vi "Process--SMO.Example.vi"(8 "error in (no error)":errorcluster, 11 "SMO.Example in":refnum<class "SMO.Example.lvclass">) -> (0 "error out":errorcluster)   [LabVIEW 2013, in "SMO.Example.lvclass"]
uses:
  SMO.Example.lvclass
  src/SMO/SMO.lvclass
panel:
  out "Flow 2":dbl
  out "Flow 1":dbl
  in  "Pump State":bool
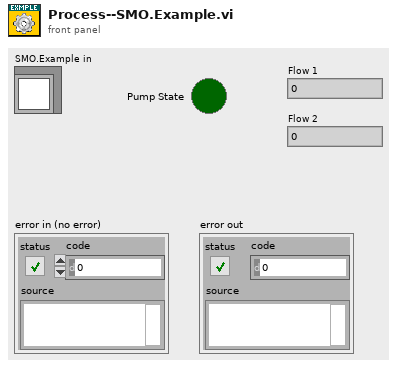
[diagram p1: front panel]
types:
  T1 = enum32{"invalid app kind", "Development System", "Run Time System", "Student Edition", "Embedded LabVIEW", "Evaluation", "Custom"}
  T2 = enum32{"Invalid", "Standard", "Closed", "Hidden", "Minimized", "Maximized"}
  T3 = cluster{"Core":cluster{"Current VI Reference":refnum<vi>, "Close Panel on Exit?":bool, "error":errorcluster, "Standalone":bool}, "Self Ref":refnum<class "SMO.Example.lvclass">, "Your string data":string, "Pump State":bool, "Valve 1 State":bool, "Flow 1 Actual":dbl, "Flow 2 Actual":dbl, "Flow 1 Target":dbl, "Flow 2 Target":dbl}
  T4 = typedef "SMO.lvclass/SMOState --Enum.ctl" = enum16{"unknown", "Created", "Started", "Stopped"}
  T5 = cluster{"Current VI Reference":refnum<vi>, "Close Panel on Exit?":bool, "error":errorcluster, "Standalone":bool}
  T6 = typedef "SMO.lvclass/Protected Events.ctl" = cluster{"StopProcesses":refnum<user-event>, "AbortProcesses":refnum<user-event>, "Config Changed":refnum<user-event>, "Dependency":refnum<user-event>}
  T7 = typedef "SMO.Example.lvclass/ProtectedEvents--Cluster.ctl" = cluster{"API_Template":refnum<user-event>, "PumpState":refnum<user-event>, "Valve State":refnum<user-event>}
  T8 = typedef "SMO.Example.lvclass/PublicEvents--Cluster.ctl" = cluster{"Data Changed":refnum<user-event>, "State Changed":refnum<user-event>}
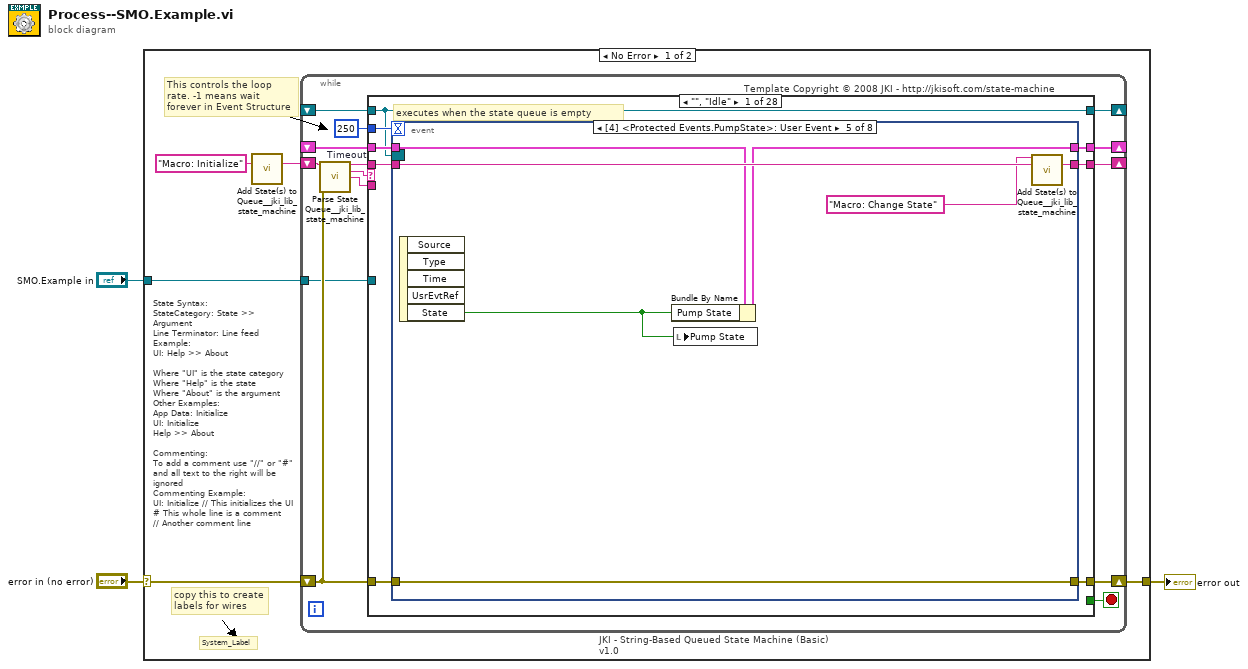
[diagram p0: block diagram]
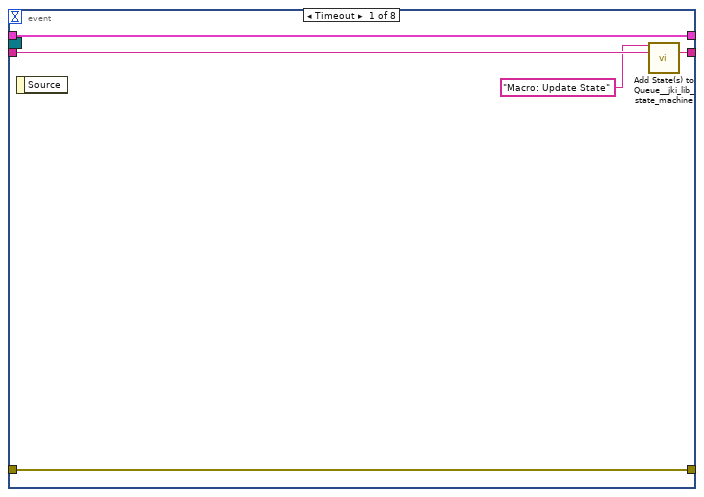
[diagram p2: hidden frame]
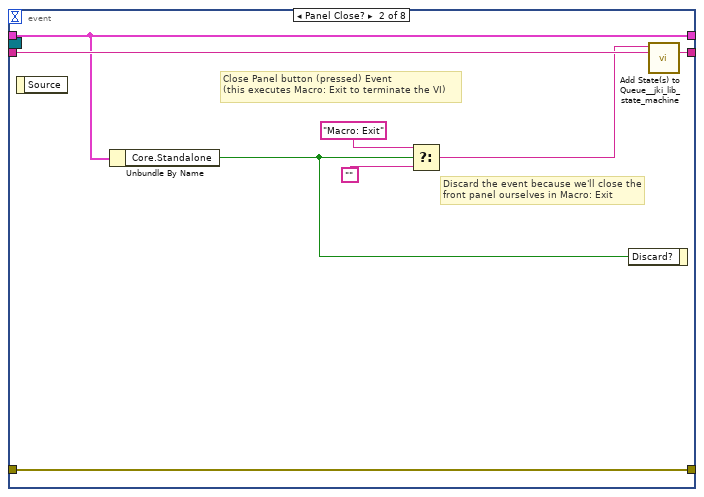
[diagram p3: hidden frame]
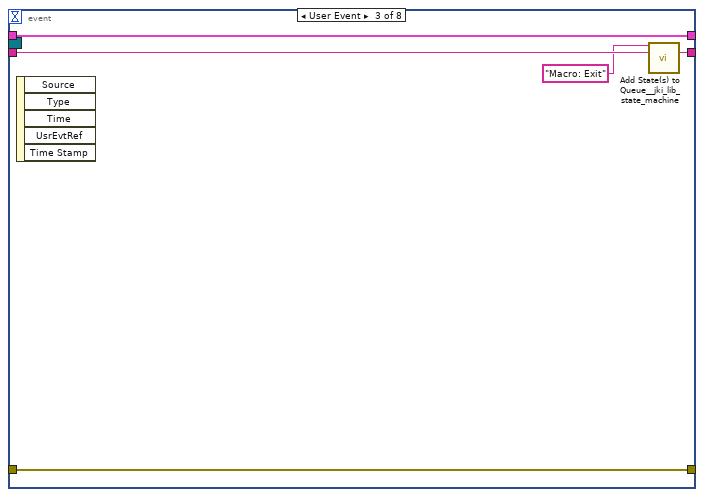
[diagram p4: hidden frame]
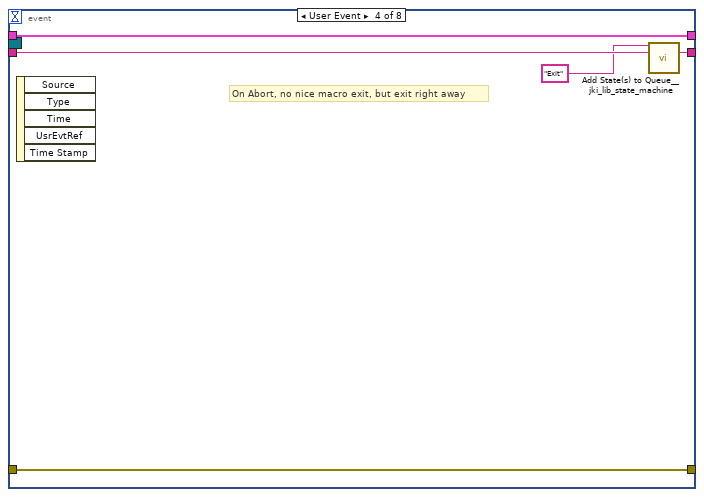
[diagram p5: hidden frame]
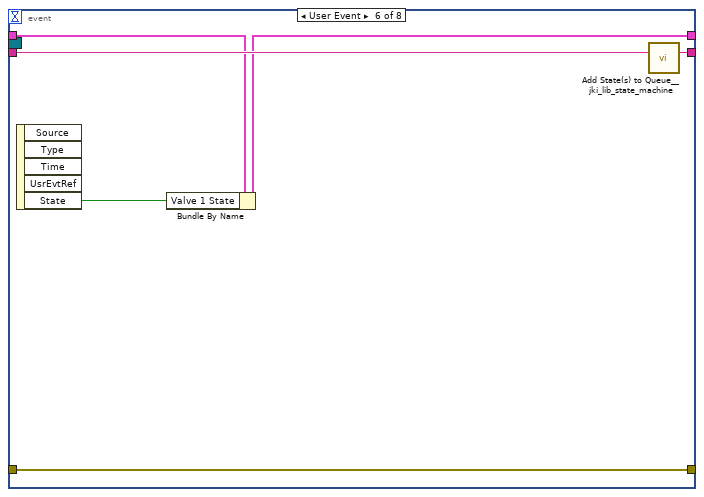
[diagram p6: hidden frame]
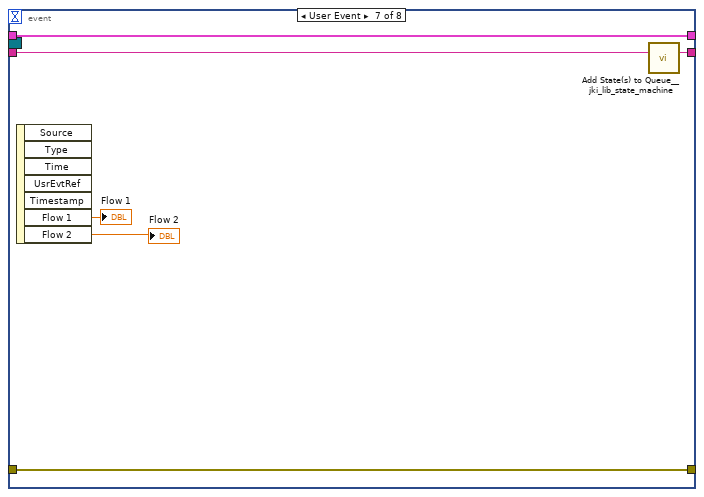
[diagram p7: hidden frame]
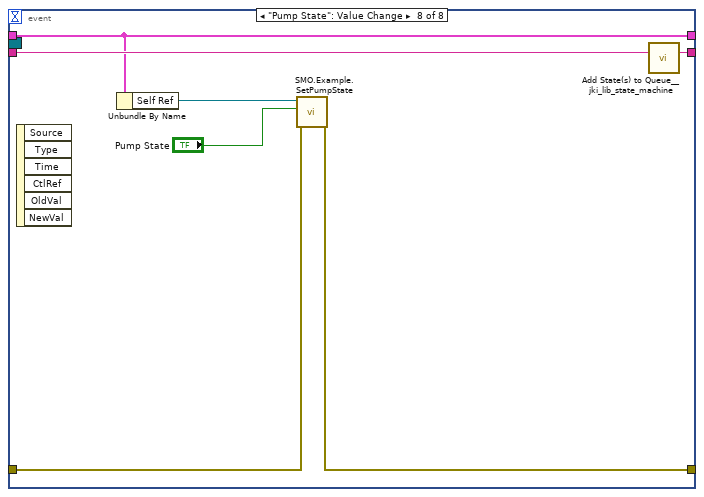
[diagram p8: hidden frame]
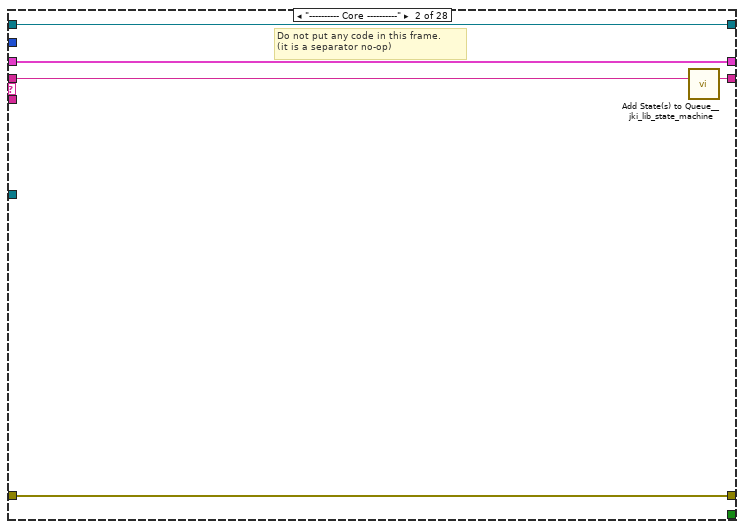
[diagram p9: hidden frame]
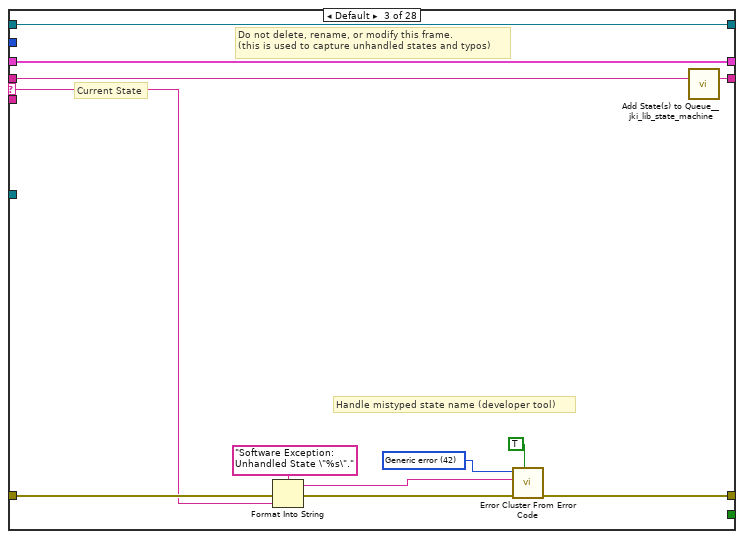
[diagram p10: hidden frame]
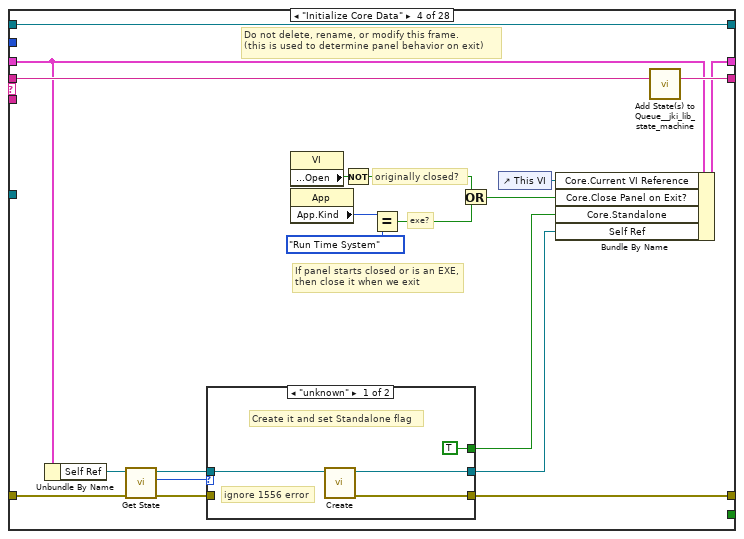
[diagram p11: hidden frame]
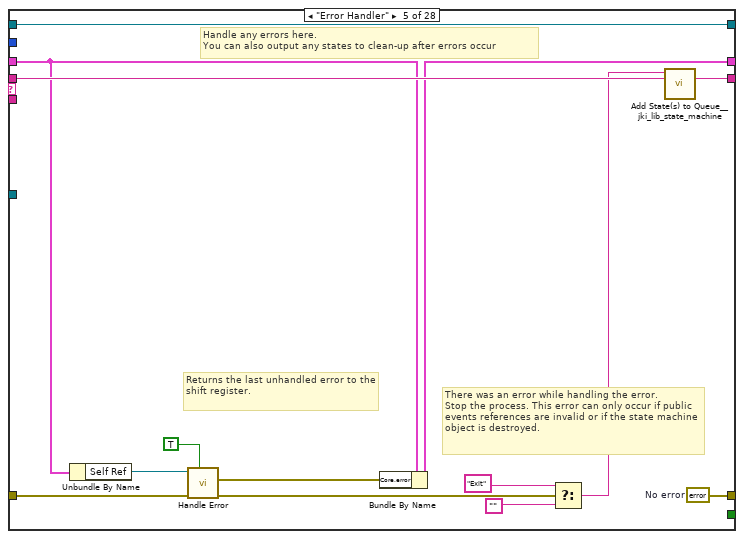
[diagram p13: hidden frame]
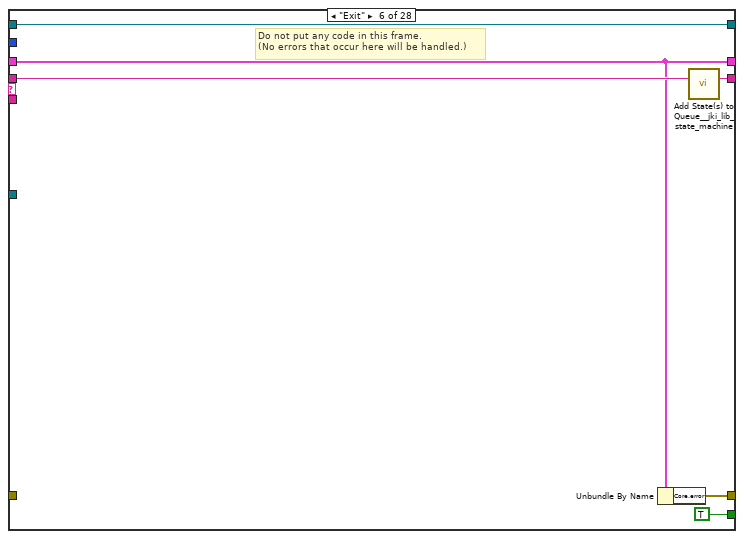
[diagram p14: hidden frame]
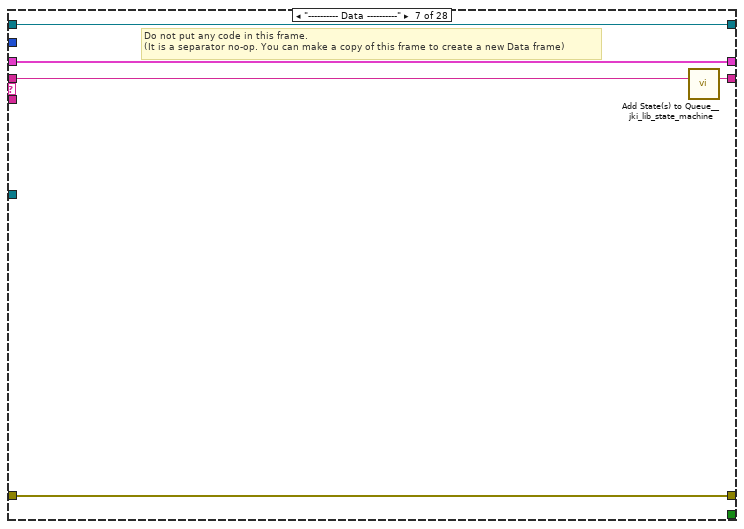
[diagram p15: hidden frame]
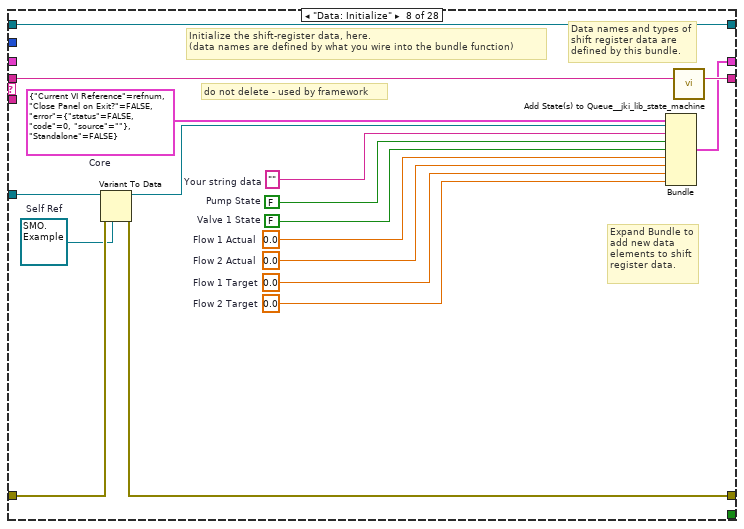
[diagram p16: hidden frame]
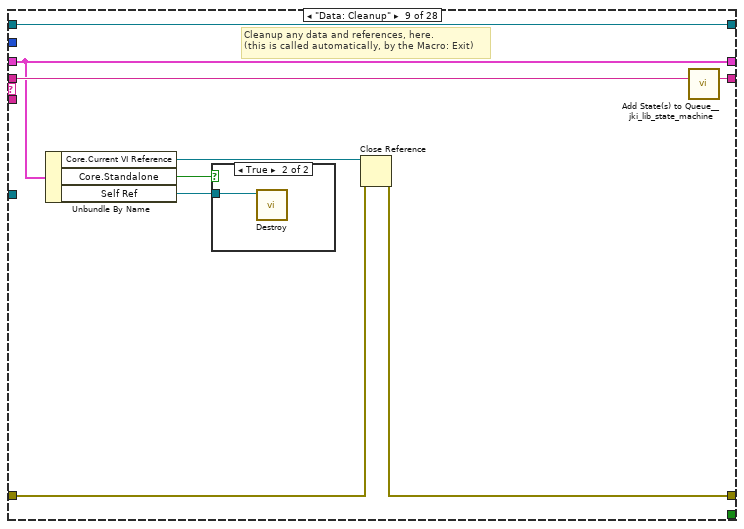
[diagram p17: hidden frame]
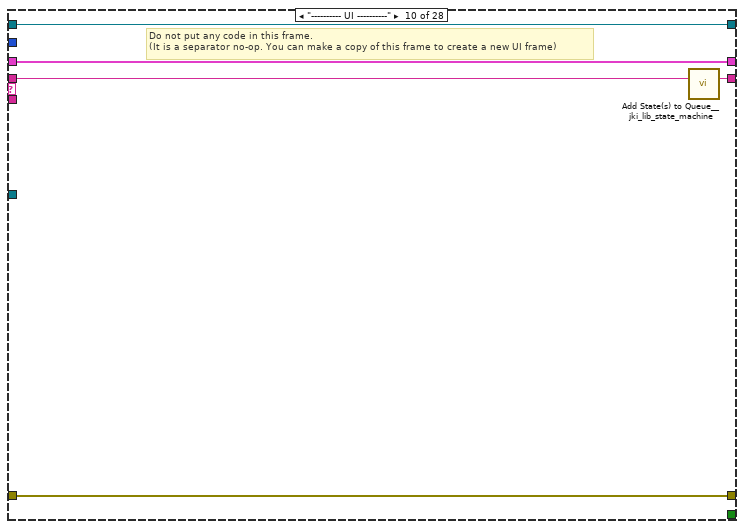
[diagram p19: hidden frame]
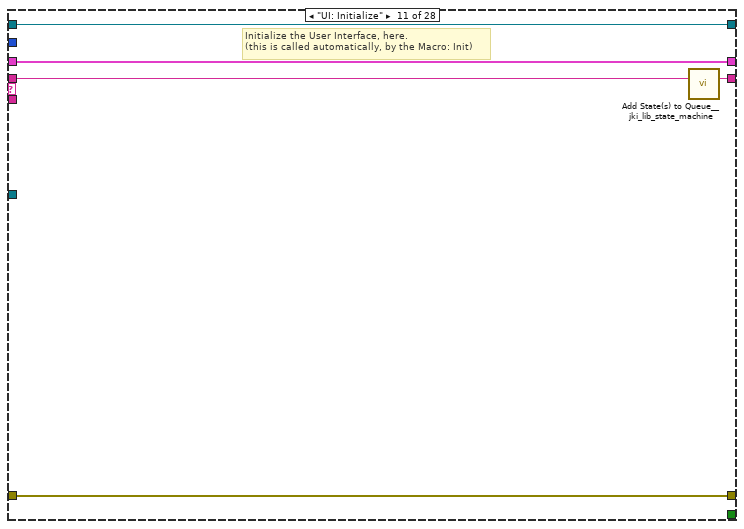
[diagram p20: hidden frame]
diagram:
  n1 = case shown="No Error" "error in (no error)" {
    selector: "error in (no error)" -> [w5 w378]
    tunnel: "SMO.Example in" -> [w6 _]
    tunnel: [w4 w378] -> w3
    frame No Error {
      # "State Syntax:\nStateCategory: State >> Argument\nLine Terminator: Line feed\nExample:\nUI: Help >> About\n\nWhere \"UI\" is the state category\nWhere \"Help\" is the state\nWhere \"About\" is the argument\nOther Examples:\nApp Data: Initialize\nUI: Initialize\nHelp >> About\n\nCommenting:\nTo add a comment use \"//\" or \"#\" and all text to the right will be ignored\nCommenting Example:\nUI: Initialize // This initializes the UI\n# This whole line is a comment\n// Another comment line"
      # "copy this to create labels for wires"
      # "This controls the loop rate. -1 means wait forever in Event Structure"
      # "System_Label"
      n2 = call <vilib>:"Add State(s) to Queue__jki_lib_state_machine.vi"("State(s) in (\"\")"="Macro: Initialize") -> ("States Out"=w8:string)  [unwired: 14 in]
      n3 = while "JKI - String-Based Queued State Machine (Basic) v1.0" {
        shift-right: [w15] -> _
        shift-left: _ -> [w14]
        shift-right: [w18] -> w4
        shift-left: w5 -> [w12]
        shift-right: [w17] -> _
        shift-left: w8 -> [w19]
        tunnel: w6 -> [w11]
        shift-right: [w10] -> _
        shift-left: _ -> [w9]
        stop <- w16 stop-if-true
        w13 = 250  # Timeout
        # "Template Copyright © 2008 JKI - http://jkisoft.com/state-machine"
        n4 = call <vilib>:"Parse State Queue__jki_lib_state_machine.vi"("State Queue"=w19, "Error In (no error)"=w12) -> ("Remaining States"=w21:string, "Current State"=w22:string, "Arguments"=w20:string)  [unwired: 11 in]
        n5 = case shown="\"\", \"Idle\"" w22 {
          selector: w22 -> [_ _ w86 _ _ _ _ _ _ _ _ _ _ _ _ _ _ _ _ _ _ _ _ _ _ _ _ _]
          tunnel: w21 -> [w30 w84 w90 w116 w136 w142 w147 w164 w173 w179 w184 w189 w197 w229 w238 w244 w250 w261 w266 w275 w288 w303 w309 w314 w324 w360 w369 w377]
          tunnel: w20 -> [_ _ _ _ _ _ _ _ _ _ _ _ w190 _ _ _ _ _ _ _ _ _ _ _ _ _ _ _]
          tunnel: w14 -> [w28 w81 w88 w104 w127 w138 w144 _ w168 w176 w182 w187 w195 w226 w234 w241 w247 w252 w263 w272 w285 w301 w307 w312 w318 w356 w366 w374]
          tunnel: [w27 w82 w92 w100 w124 w137 w145 w159 w169 w177 w181 w185 w191 w227 w236 w242 w248 w259 w264 w269 w286 w295 w305 w310 w319 w357 w363 w370] -> w18
          tunnel: w12 -> [w26 w82 w91 w103 w128 _ w145 w160 w170 w177 w181 w185 w192 w227 w236 w242 w248 w259 w264 w270 w286 w297 w305 w310 w319 w357 w364 w371]
          tunnel: [w29 w83 w89 w115 w135 w141 w146 w163 w172 w178 w183 w188 w196 w228 w237 w243 w249 w260 w265 w274 w287 w302 w308 w313 w323 w359 w368 w376] -> w17
          tunnel: [_ _ _ _ _ TRUE _ _ _ _ _ _ _ _ _ _ _ _ _ _ _ _ _ _ _ _ _ _] -> w16
          tunnel: [w25 w81 w88 w114 w126 w138 w144 w162 w168 w176 w182 w187 w195 w226 w234 w241 w247 w252 w263 w272 w285 w301 w307 w312 w317 w355 w366 w374] -> w15
          tunnel: w13 -> [w24 _ _ _ _ _ _ _ _ _ _ _ _ _ _ _ _ _ _ _ _ _ _ _ _ _ _ _]
          tunnel: w11 -> [_ _ _ _ _ _ _ w157 _ _ _ _ _ _ _ _ _ _ _ _ _ _ _ _ _ _ _ _]
          tunnel: [w23 w80 w85 w107 w134 w139 w143 w155 w167 w175 w180 w186 w194 w225 w235 w240 w246 w253 w262 w273 w284 w299 w306 w311 w322 w358 w367 w375] -> w10
          tunnel: w9 -> [w23 w80 w85 w107 w134 w139 w143 w155 w167 w175 w180 w186 w194 w225 w235 w240 w246 w253 w262 w273 w284 _ w306 w311 w322 w358 w367 w375]
          frame "", "Idle" {
            # "executes when the state queue is empty"
            n6 = event shown="[4] <Protected Events.PumpState>: User Event" {
              selector: w23 -> [_ _ _ _ _ _ _ _]
              dyn-events: _ -> [_ _ _ _ _ _ _ _]
              timeout: w24 -> [_ _ _ _ _ _ _ _]
              tunnel: w30 -> [w35 w43 w48 w53 w60 w66 w72 w79]
              tunnel: [w34 w42 w47 w52 w59 w65 w71 w78] -> w29
              tunnel: w28 -> [w32 w40 w45 w50 w57 w63 w69 w77]
              tunnel: [w33 w41 w46 w51 w58 w64 w70 w73] -> w27
              tunnel: w26 -> [w33 w41 w46 w51 w58 w64 w70 w74]
              tunnel: [w32 w40 w45 w50 w56 w62 w69 w77] -> w25
              event Timeout {
                n7 = event-data() -> ()  [unwired: 1 in, 1 out]
                n8 = call <vilib>:"Add State(s) to Queue__jki_lib_state_machine.vi"("State(s) in Front (\"\")"="Macro: Update State", "State(s) in (\"\")"=w35) -> ("States Out"=w34:string)  [unwired: 13 in]
              }
              event Panel Close? {
                # "Discard the event because we'll close the front panel ourselves in Macro: Exit"
                # "Close Panel button (pressed) Event\n(this executes Macro: Exit to terminate the VI)"
                n9 = event-data() -> ()  [unwired: 1 in, 1 out]
                n10 = Unbundle By Name(w40) -> ("Core.Standalone"=w36:bool)
                n11 = Select(t="Macro: Exit", s=w36, f="") -> (s? t:f=w37:string)
                n12 = event-data("Discard?"=w36) -> ()  [unwired: 1 in, 1 out]
                n13 = call <vilib>:"Add State(s) to Queue__jki_lib_state_machine.vi"("State(s) in Front (\"\")"=w37, "State(s) in (\"\")"=w43) -> ("States Out"=w42:string)  [unwired: 13 in]
              }
              event User Event {
                n14 = event-data() -> ()  [unwired: 1 in, 5 out]
                n15 = call <vilib>:"Add State(s) to Queue__jki_lib_state_machine.vi"("State(s) in Front (\"\")"="Macro: Exit", "State(s) in (\"\")"=w48) -> ("States Out"=w47:string)  [unwired: 13 in]
              }
              event User Event {
                # "On Abort, no nice macro exit, but exit right away"
                n16 = event-data() -> ()  [unwired: 1 in, 5 out]
                n17 = call <vilib>:"Add State(s) to Queue__jki_lib_state_machine.vi"("State(s) in Front (\"\")"="Exit", "State(s) in (\"\")"=w53) -> ("States Out"=w52:string)  [unwired: 13 in]
              }
              event User Event {
                n18 = event-data() -> ("State"=w54:bool)  [unwired: 1 in, 4 out]
                n19 = Bundle By Name(cluster=w57, "Pump State"=w54) -> (w56:T3)
                n20 = local write "Pump State"(w54) -> ()
                n21 = call <vilib>:"Add State(s) to Queue__jki_lib_state_machine.vi"("State(s) in Front (\"\")"="Macro: Change State", "State(s) in (\"\")"=w60) -> ("States Out"=w59:string)  [unwired: 13 in]
              }
              event User Event {
                n22 = event-data() -> ("State"=w61:bool)  [unwired: 1 in, 4 out]
                n23 = Bundle By Name(cluster=w63, "Valve 1 State"=w61) -> (w62:T3)
                n24 = call <vilib>:"Add State(s) to Queue__jki_lib_state_machine.vi"("State(s) in (\"\")"=w66) -> ("States Out"=w65:string)  [unwired: 14 in]
              }
              event User Event {
                n25 = event-data() -> ("Flow 1"=→"Flow 1":dbl, "Flow 2"=→"Flow 2":dbl)  [unwired: 1 in, 5 out]
                n26 = call <vilib>:"Add State(s) to Queue__jki_lib_state_machine.vi"("State(s) in (\"\")"=w72) -> ("States Out"=w71:string)  [unwired: 14 in]
              }
              event "Pump State": Value Change {
                n27 = event-data() -> ()  [unwired: 1 in, 6 out]
                n28 = Unbundle By Name(w77) -> ("Self Ref"=w76:refnum<class "SMO.Example.lvclass">)
                n29 = call "SMO.Example.SetPumpState.vi"("error in (no error)"=w74, "Pump State"="Pump State", "SMO.Example"=w76) -> ("error out"=w73:errorcluster)  [unwired: 7 in, 1 out]
                n30 = call <vilib>:"Add State(s) to Queue__jki_lib_state_machine.vi"("State(s) in (\"\")"=w79) -> ("States Out"=w78:string)  [unwired: 14 in]
              }
            }
          }
          frame "---------- Core ----------" {
            # "Do not put any code in this frame.\n(it is a separator no-op)"
            n31 = call <vilib>:"Add State(s) to Queue__jki_lib_state_machine.vi"("State(s) in (\"\")"=w84) -> ("States Out"=w83:string)  [unwired: 14 in]
          }
          frame Default {
            w95 = 42 items=["No error", "Argument error", "Memory is full", "Out of zone", "End of file", "File already open", "Generic file I/O error", "File not found", "File permission error", "Disk is full", "Duplicate path", "Too many files open", "System feature not enabled", "Resource file not found", "Cannot add resource", "Resource not found", "Image not found", "Image memory error", "Pen does not exist", "Config type invalid", "Config token not found", "Config parse error", "Config memory error", "Bad external code format", "Bad external code offset", "External code not present", "Null window", "Destroy window error", "Null menu", "Print aborted", "Bad print record", "Print driver error", "Windows error during printing", "Memory error during printing", "Print dialog error", "Generic print error", "Invalid device refnum", "Device not found", "Device parameter error", "Device unit error", "Cannot open device", "Device call aborted", "Generic error", "Cancelled by user", "Object ID too low", "Object ID too high", "Object not in heap", "Unknown heap", "Unknown object (invalid DefProc)", "Unknown object (DefProc not in table)", "Message out of range", "Invalid (null) method", "Unknown message", "Manager call not supported", "Bad address", "Network operation in progress", "Network operation timed out", "Connection is busy", "Network attribute not supported", "Network error", "Address in use", "System out of memory", "Connection aborted", "Connection refused", "Not connected", "Already connected", "Connection closed", "Initialization error (interapplication manager)", "Bad occurrence", "Wait on unbound occurrence handler", "Occurrence queue overflow", "Datalog type conflict", "Unused", "Unrecognized type (interapplication manager)", "Memory corrupt", "Failed to make temporary DLL", "Old CIN version", "Drag socket not found", "Failed to load drop-object", "Failed to register OLE object", "Failed to release OLE object", "Format specifier type mismatch", "Unknown format specifier", "Too few format specifiers", "Too many format specifiers", "Scan failed", "Newer CIN version", "Error converting to variant", "Runtime menu error", "Password tampered", "Variant attribute not found", "Incompatible variant data type", "Event data is not available", "Event Store is not present", "Occurrence is not found", "Event Queue is not created", "Event info is not available", "Refnum passed is NULL", "Error retrieving Class GUID", "Error retrieving CoClass GUID", "Error retrieving TypeLib GUID.", "Bad built application magic bytes.", "Specific driver is different from the specific driver associated with the Logical Name.", "There is no session opened to the class driver.", "Max Error", "MAX - Error with config objects", "MAX - Error loading configuration", "MAX - Group not supported"]
            # "Current State"
            # "Do not delete, rename, or modify this frame.\n(this is used to capture unhandled states and typos)"
            # "Handle mistyped state name (developer tool)"
            n32 = Format Into String(format string="Software Exception: Unhandled State \"%s\"." ("message"), error in=w91, w86) -> (resulting string=w94:string, error out=w93:errorcluster)  [unwired: 1 in]
            n33 = call <vilib>:"Error Cluster From Error Code.vi"("show call chain? (False)"=TRUE, "error in (no error)"=w93, "error message (\"\")"=w94, "error code (0)"=w95) -> ("error out"=w92:errorcluster)  [unwired: 5 in]
            n34 = call <vilib>:"Add State(s) to Queue__jki_lib_state_machine.vi"("State(s) in (\"\")"=w90) -> ("States Out"=w89:string)  [unwired: 14 in]
          }
          frame "Initialize Core Data" {
            # "Do not delete, rename, or modify this frame.\n(this is used to determine panel behavior on exit)"
            # "originally closed?"
            # "exe?"
            # "If panel starts closed or is an EXE, then close it when we exit"
            n35 = Unbundle By Name(w104) -> ("Self Ref"=w105:refnum<class "SMO.Example.lvclass">)
            n36 = call "Get State.vi"("error in (no error)"=w103, "SMO"=w105) -> ("error out"=w101:errorcluster, "SMO State"=w102:T4, "SMO out"=w98:refnum<class "SMO.Example.lvclass">)  [unwired: 7 in]
            n37 = case shown="\"unknown\"" w102 {
              tunnel: w101 -> [_ w122]
              tunnel: [w119 w122] -> w100
              tunnel: [TRUE _] -> w99
              tunnel: w98 -> [w118 w121]
              tunnel: [w117 w121] -> w97
              frame "unknown" {
                # "ignore 1556 error"
                # "Create it and set Standalone flag"
                n38 = call "Create.vi"("SMO"=w118) -> ("error out"=w119:errorcluster, "SMO out"=w117:refnum<class "SMO.Example.lvclass">)  [unwired: 8 in, 1 out]
              }
              frame Default {
              }
            }
            n39 = property class="VI"() -> ("Front Panel.Open"=w113:bool)  [unwired: 2 in, 2 out]
            n40 = property class="App"() -> ("App.Kind"=w112:T1)  [unwired: 2 in, 2 out]
            n41 = Not(x=w113) -> (.not. x?=w110:bool)
            n42 = Equal?(x=w112, y=T1."Run Time System" ("Application:Kind")) -> (x = y?=w109:bool)
            n43 = Or(x=w110, y=w109) -> (x .or. y?=w108:bool)
            n44 = control-ref of="This VI"() -> (w106:refnum<vi>)
            n45 = Bundle By Name(cluster=w104, "Core.Current VI Reference"=w106, "Core.Close Panel on Exit?"=w108, "Core.Standalone"=w99, "Self Ref"=w97) -> (w114:T3)
            n46 = call <vilib>:"Add State(s) to Queue__jki_lib_state_machine.vi"("State(s) in (\"\")"=w116) -> ("States Out"=w115:string)  [unwired: 14 in]
          }
          frame "Error Handler" {
            w124 = errorcluster {"status"=FALSE, "code"=0, "source"=""}  # No error
            # "Returns the last unhandled error to the shift register."
            # "There was an error while handling the error.\nStop the process. This error can only occur if public events references are invalid or if the state machine object is destroyed."
            # "Handle any errors here.\nYou can also output any states to clean-up after errors occur"
            n47 = Unbundle By Name(w127) -> ("Self Ref"=w129:refnum<class "SMO.Example.lvclass">)
            n48 = call-dynamic "Handle Error.vi"("Stop on Unhandled Error (T)"=TRUE, "error in"=w128, "SMO"=w129) -> ("handling error"=w131:errorcluster, "Unhandled error"=w130:errorcluster)  [unwired: 6 in, 1 out]
            n49 = Bundle By Name(cluster=w127, "Core.error"=w130) -> (w126:T3)
            n50 = Select(t="Exit", s=w131, f="") -> (s? t:f=w125:string)
            n51 = call <vilib>:"Add State(s) to Queue__jki_lib_state_machine.vi"("State(s) in Front (\"\")"=w125, "State(s) in (\"\")"=w136) -> ("States Out"=w135:string)  [unwired: 13 in]
          }
          frame "Exit" {
            # "Do not put any code in this frame.\n(No errors that occur here will be handled.)"
            n52 = Unbundle By Name(w138) -> ("Core.error"=w137:errorcluster)
            n53 = call <vilib>:"Add State(s) to Queue__jki_lib_state_machine.vi"("State(s) in (\"\")"=w142) -> ("States Out"=w141:string)  [unwired: 14 in]
          }
          frame "---------- Data ----------" {
            # "Do not put any code in this frame.\n(It is a separator no-op. You can make a copy of this frame to create a new Data frame)"
            n54 = call <vilib>:"Add State(s) to Queue__jki_lib_state_machine.vi"("State(s) in (\"\")"=w147) -> ("States Out"=w146:string)  [unwired: 14 in]
          }
          frame "Data: Initialize" {
            w148 = T5 {"Current VI Reference"=refnum, "Close Panel on Exit?"=FALSE, "error"={"status"=FALSE, "code"=0, "source"=""}, "Standalone"=FALSE}  # Core
            w149 = 0.0  # Flow 2 Target
            w150 = 0.0  # Flow 1 Target
            w151 = 0.0  # Flow 2 Actual
            w152 = 0.0  # Flow 1 Actual
            w153 = FALSE  # Valve 1 State
            w154 = FALSE  # Pump State
            w158 = refnum<class "SMO.Example.lvclass"> refnum  # Self Ref
            w161 = ""  # Your string data
            # "do not delete - used by framework"
            # "Expand Bundle to add new data elements to shift register data."
            # "Data names and types of shift register data are defined by this bundle."
            # "Initialize the shift-register data, here.\n(data names are defined by what you wire into the bundle function)"
            n55 = Variant To Data(error in=w160, type=w158, Variant=w157) -> (data=w156:refnum<class "SMO.Example.lvclass">, error out=w159:errorcluster)
            n56 = Bundle("Core"=w148, "Self Ref"=w156, "Your string data"=w161, "Pump State"=w154, "Valve 1 State"=w153, "Flow 1 Actual"=w152, "Flow 2 Actual"=w151, "Flow 1 Target"=w150, "Flow 2 Target"=w149) -> (w162:T3)  [unwired: 1 in]
            n57 = call <vilib>:"Add State(s) to Queue__jki_lib_state_machine.vi"("State(s) in (\"\")"=w164) -> ("States Out"=w163:string)  [unwired: 14 in]
          }
          frame "Data: Cleanup" {
            # "Cleanup any data and references, here.\n(this is called automatically, by the Macro: Exit)"
            n58 = Unbundle By Name(w168) -> ("Core.Current VI Reference"=w171:refnum<vi>, "Core.Standalone"=w166:bool, "Self Ref"=w165:refnum<class "SMO.Example.lvclass">)
            n59 = case shown="True" w166 {
              tunnel: w165 -> [_ w174]
              frame False {
              }
              frame True {
                n60 = call "Destroy.vi"("SMO"=w174) -> ()  [unwired: 10 in, 1 out]
              }
            }
            n61 = Close Reference(reference=w171, error in (no error)=w170) -> (error out=w169:errorcluster)
            n62 = call <vilib>:"Add State(s) to Queue__jki_lib_state_machine.vi"("State(s) in (\"\")"=w173) -> ("States Out"=w172:string)  [unwired: 14 in]
          }
          frame "---------- UI ----------" {
            # "Do not put any code in this frame.\n(It is a separator no-op. You can make a copy of this frame to create a new UI frame)"
            n63 = call <vilib>:"Add State(s) to Queue__jki_lib_state_machine.vi"("State(s) in (\"\")"=w179) -> ("States Out"=w178:string)  [unwired: 14 in]
          }
          frame "UI: Initialize" {
            # "Initialize the User Interface, here.\n(this is called automatically, by the Macro: Init)"
            n64 = call <vilib>:"Add State(s) to Queue__jki_lib_state_machine.vi"("State(s) in (\"\")"=w184) -> ("States Out"=w183:string)  [unwired: 14 in]
          }
          frame "UI: Cursor Set" {
            # "Deleted Cursor Busy code\nto make process RT-compatible"
            # "Initialize the User Interface, here.\n(this is called automatically, by the Macro: Init)"
            n65 = call <vilib>:"Add State(s) to Queue__jki_lib_state_machine.vi"("State(s) in (\"\")"=w189) -> ("States Out"=w188:string)  [unwired: 14 in]
          }
          frame "UI: Front Panel State" {
            # "Argument"
            # "Set Front Panel Open or Closed\n(Usage: \"UI: Front Panel State >> Open|Close\")"
            n66 = Unbundle By Name(w195) -> ("Core.Current VI Reference"=w193:refnum<vi>)
            n67 = disable-structure shown="Default" {
              disable-tunnel: w192 -> [w201 w224]
              disable-tunnel: [w200 w224] -> w191
              disable-tunnel: w193 -> [w199 _]
              disable-tunnel: w190 -> [w198 _]
              frame condition #0 (active) {
                n68 = case shown="\"Open\"" w198 {
                  tunnel: w201 -> [w205 w218]
                  tunnel: [w207 w219] -> w200
                  tunnel: w199 -> [w206 w216]
                  frame "Open" {
                    # "Open FP if not open or invalid"
                    n69 = property class="VI"(reference=w206, error in=w205) -> (reference out=w203:refnum<vi>, error out=w204:errorcluster, "FP.State"=w202:T2)
                    n70 = case shown="Default" w202 {
                      tunnel: [w210 w213] -> w207
                      tunnel: w204 -> [w209 w213]
                      tunnel: w203 -> [w208 _]
                      frame Default {
                        n71 = invoke class="VI" method="FP.Open"(reference=w208, error in=w209, "Activate"=TRUE, "State"=T2."Standard") -> (error out=w210:errorcluster)  [unwired: 1 in, 4 out]
                      }
                      frame "Invalid", "Standard" {
                      }
                    }
                  }
                  frame "Close", Default {
                    # "Close FP is not Closed or Invalid"
                    n72 = property class="VI"(reference=w216, error in=w218) -> (reference out=w215:refnum<vi>, error out=w217:errorcluster, "FP.State"=w214:T2)
                    n73 = case shown="Default" w214 {
                      tunnel: [w220 w223] -> w219
                      tunnel: w217 -> [w220 w222]
                      tunnel: w215 -> [_ w221]
                      frame "Invalid", "Closed" {
                      }
                      frame Default {
                        n74 = invoke class="VI" method="FP.Close"(reference=w221, error in=w222) -> (error out=w223:errorcluster)  [unwired: 1 in, 2 out]
                      }
                    }
                  }
                }
              }
              frame condition #1 {
              }
            }
            n75 = call <vilib>:"Add State(s) to Queue__jki_lib_state_machine.vi"("State(s) in (\"\")"=w197) -> ("States Out"=w196:string)  [unwired: 14 in]
          }
          frame "---------- Macro ----------" {
            # "Do not put any code in this frame.\n(It is a separator no-op. You can make a copy of this frame to create a new Macro frame)"
            n76 = call <vilib>:"Add State(s) to Queue__jki_lib_state_machine.vi"("State(s) in (\"\")"=w229) -> ("States Out"=w228:string)  [unwired: 14 in]
          }
          frame "Macro: Initialize" {
            w232 = "UI: Initialize\n//UI: Front Panel State >> Open"  # UI: Initialize //UI: Front Panel State >> Open
            # "Initialization Macro\n(This is called once, when the VI starts)"
            n77 = call <vilib>:"Add State(s) to Queue__jki_lib_state_machine.vi"("State(s) in Front (\"\")"="Data: Initialize\nInitialize Core Data\nEvents: Register", "State(s) in (\"\")"="Process: Sync", "State(s) at Back (\"\")"=w232) -> ("States Out"=w231:string)  [unwired: 12 in]
            n78 = call <vilib>:"Add State(s) to Queue__jki_lib_state_machine.vi"("State(s) in Front (\"\")"=w231, "State(s) in (\"\")"=w238) -> ("States Out"=w237:string)  [unwired: 13 in]
          }
          frame "Macro: Update State" {
            n79 = call <vilib>:"Add State(s) to Queue__jki_lib_state_machine.vi"("State(s) in Front (\"\")"="Action: Determine Flow Targets\nAction: Determine Actual Flow\nAction: Update State", "State(s) in (\"\")"=w244) -> ("States Out"=w243:string)  [unwired: 13 in]
          }
          frame "Macro: Change State" {
            n80 = call <vilib>:"Add State(s) to Queue__jki_lib_state_machine.vi"("State(s) in Front (\"\")"="Action: Change State\nAction: Update State", "State(s) in (\"\")"=w250) -> ("States Out"=w249:string)  [unwired: 13 in]
          }
          frame "Macro: Exit" {
            # "Exit Macro\n(This is called once, when the VI exits)"
            n81 = Unbundle By Name(w252) -> ("Core.Close Panel on Exit?"=w258:bool)
            n82 = Select(t="//UI: Front Panel State >> Close", s=w258, f="") -> (s? t:f=w255:string)
            n83 = call <vilib>:"Add State(s) to Queue__jki_lib_state_machine.vi"("State(s) in (\"\")"=w255, "State(s) at Back (\"\")"="Data: Cleanup\nEvents: Unregister\nProcess: Sync\nExit") -> ("States Out"=w254:string)  [unwired: 13 in]
            n84 = call <vilib>:"Add State(s) to Queue__jki_lib_state_machine.vi"("State(s) in Front (\"\")"=w254, "State(s) in (\"\")"=w261) -> ("States Out"=w260:string)  [unwired: 13 in]
          }
          frame "---------- Process ----------" {
            # "Template Separator\n(You can make a copy of, or modify, this frame)"
            n85 = call <vilib>:"Add State(s) to Queue__jki_lib_state_machine.vi"("State(s) in (\"\")"=w266) -> ("States Out"=w265:string)  [unwired: 14 in]
          }
          frame "Process: Sync" {
            # "Synchronizing Processes\nStarting and Stopping Processes needs to be synchronized"
            n86 = Unbundle By Name(w272) -> ("Core.Standalone"=w267:bool, "Self Ref"=w271:refnum<class "SMO.Example.lvclass">)
            n87 = case shown="False" w267 {
              tunnel: w271 -> [w279 _]
              tunnel: w270 -> [w278 w283]
              tunnel: [w277 w283] -> w269
              tunnel: [w276 _] -> w268
              frame False {
                n88 = call "WaitOnProcessSync.vi"("error in (no error)"=w278, "SMO"=w279) -> ("error out"=w277:errorcluster, "Don't run?"=w282:bool)  [unwired: 7 in, 1 out]
                n89 = Select(t="Data: Cleanup\nEvents: Unregister\nExit", s=w282, f="") -> (s? t:f=w276:string)
              }
              frame True {
              }
            }
            n90 = call <vilib>:"Add State(s) to Queue__jki_lib_state_machine.vi"("State(s) in Front (\"\")"=w268, "State(s) in (\"\")"=w275) -> ("States Out"=w274:string)  [unwired: 13 in]
          }
          frame "---------- Events ----------" {
            # "Template Separator\n(You can make a copy of, or modify, this frame)"
            n91 = call <vilib>:"Add State(s) to Queue__jki_lib_state_machine.vi"("State(s) in (\"\")"=w288) -> ("States Out"=w287:string)  [unwired: 14 in]
          }
          frame "Events: Register" {
            # "Self Public Events >>"
            # "Self Protected Events >>"
            # "Base Class Protected Events"
            # "Register Events here."
            n92 = Unbundle By Name(w301) -> ("Self Ref"=w291:refnum<class "SMO.Example.lvclass">)
            n93 = call "GetProtectedEvents.vi"("SMO"=w291) -> ("error out"=w294:errorcluster, "SMO Protected Events"=w300:T6)  [unwired: 8 in, 1 out]
            n94 = call "SMO.Example.GetProtectedEvents.vi"("SMO.Example"=w291) -> ("error out"=w293:errorcluster, "Protected Events"=w298:T7)  [unwired: 8 in, 1 out]
            n95 = call "SMO.Example.GetPublicEvents.vi"("SMO.Example"=w291) -> ("error out"=w289:errorcluster, "SMO.Example Public Events"=w290:T8)  [unwired: 7 in, 2 out]
            n96 = Merge Errors(w294, w293, w289) -> (w292:errorcluster)
            n97 = register-events(w300, w298, w290) -> (reference out=w299:refnum<event-registration>, error out=w296:errorcluster)  [unwired: 2 in]
            n98 = Merge Errors(w297, w296, w292) -> (w295:errorcluster)
            n99 = call <vilib>:"Add State(s) to Queue__jki_lib_state_machine.vi"("State(s) in (\"\")"=w303) -> ("States Out"=w302:string)  [unwired: 14 in]
          }
          frame "Events: Unregister" {
            n100 = Unregister For Events(event registration refnum=w306, error in=w305) -> (error out=w304:errorcluster)
            n101 = call <vilib>:"Clear Errors.vi"("error in (no error)"=w304) -> ()  [unwired: 6 in, 1 out]
            n102 = call <vilib>:"Add State(s) to Queue__jki_lib_state_machine.vi"("State(s) in (\"\")"=w309) -> ("States Out"=w308:string)  [unwired: 14 in]
          }
          frame "---------- Action ----------" {
            n103 = call <vilib>:"Add State(s) to Queue__jki_lib_state_machine.vi"("State(s) in (\"\")"=w314) -> ("States Out"=w313:string)  [unwired: 14 in]
          }
          frame "Action: Determine Flow Targets" {
            n104 = Unbundle By Name(w318) -> ("Pump State"=w321:bool, "Valve 1 State"=w320:bool)
            n105 = case "Pump On?" shown="True" w321 {
              tunnel: [w325 w329] -> w316
              tunnel: [w326 w328] -> w315
              tunnel: w320 -> [_ w332]
              frame False {
                w326 = 0.0  # Flow 2
                w325 = 0.0  # Flow 1
                # "If Pump is OFF, simulate no flow for either meter"
              }
              frame True {
                # "Simulated flow setpoint data"
                n106 = Select(t=9.0, s=w332, f=0.0) -> (s? t:f=w328:dbl)
                n107 = Subtract(x=20.0, y=w328) -> (x-y=w329:dbl)
              }
            }
            n108 = Bundle By Name(cluster=w318, "Flow 1 Target"=w316, "Flow 2 Target"=w315) -> (w317:T3)
            n109 = call <vilib>:"Add State(s) to Queue__jki_lib_state_machine.vi"("State(s) in (\"\")"=w324) -> ("States Out"=w323:string)  [unwired: 14 in]
          }
          frame "Action: Determine Actual Flow" {
            # "asymptotically appraoch target value with each iteration"
            # "If target value for either is 0, don't add noise to that particular channel."
            # "Simulate flow rate data"
            n110 = Unbundle By Name(w356) -> ("Flow 1 Target"=w344:dbl, "Flow 1 Actual"=w345:dbl, "Flow 2 Target"=w333:dbl, "Flow 2 Actual"=w343:dbl)
            n111 = Equal To 0?(x=w344) -> (x = 0?=w337:bool)
            n112 = Equal To 0?(x=w333) -> (x = 0?=w341:bool)
            n113 = Random Number (0-1)() -> (number: 0 to 1=w338:dbl)
            n114 = Random Number (0-1)() -> (number: 0 to 1=w340:dbl)
            n115 = Select(t=0.0, s=w337, f=w338) -> (s? t:f=w335:dbl)
            n116 = Select(t=0.0, s=w341, f=w340) -> (s? t:f=w334:dbl)
            n117 = Subtract(x=w344, y=w345) -> (x-y=w354:dbl)
            n118 = Subtract(x=w333, y=w343) -> (x-y=w349:dbl)
            n119 = Divide(x=w354, y=4.0) -> (x/y=w352:dbl)
            n120 = Divide(x=w349, y=3.0) -> (x/y=w347:dbl)
            n121 = Add(x=w345, y=w352) -> (x+y=w351:dbl)
            n122 = Add(x=w343, y=w347) -> (x+y=w342:dbl)
            n123 = Add(x=w335, y=w351) -> (x+y=w350:dbl)
            n124 = Add(x=w342, y=w334) -> (x+y=w346:dbl)
            n125 = Bundle By Name(cluster=w356, "Flow 1 Actual"=w350, "Flow 2 Actual"=w346) -> (w355:T3)
            n126 = call <vilib>:"Add State(s) to Queue__jki_lib_state_machine.vi"("State(s) in (\"\")"=w360) -> ("States Out"=w359:string)  [unwired: 14 in]
          }
          frame "Action: Update State" {
            n127 = Unbundle By Name(w366) -> ("Self Ref"=w365:refnum<class "SMO.Example.lvclass">, "Flow 1 Actual"=w362:dbl, "Flow 2 Actual"=w361:dbl)
            n128 = call "SMO.Example.SetData.vi"("error in (no error)"=w364, "Flow 2"=w361, "Flow 1"=w362, "SMO.Example"=w365) -> ("error out"=w363:errorcluster)  [unwired: 6 in, 1 out]
            n129 = call <vilib>:"Add State(s) to Queue__jki_lib_state_machine.vi"("State(s) in (\"\")"=w369) -> ("States Out"=w368:string)  [unwired: 14 in]
          }
          frame "Action: Change State" {
            n130 = Unbundle By Name(w374) -> ("Self Ref"=w373:refnum<class "SMO.Example.lvclass">, "Pump State"=w372:bool)
            n131 = call "SMO.Example.SetState.vi"("error in (no error)"=w371, "Pump State"=w372, "SMO.Example"=w373) -> ("error out"=w370:errorcluster)  [unwired: 7 in, 1 out]
            n132 = call <vilib>:"Add State(s) to Queue__jki_lib_state_machine.vi"("State(s) in (\"\")"=w377) -> ("States Out"=w376:string)  [unwired: 14 in]
          }
        }
      }
    }
    frame Error {
    }
  }
  "error out" <- w3
